vi "Read Tab Control Pane Dimension Width.vi"(8 "error in (no error)":errorcluster, 11 "TabControl.lvclass in":refnum<class "TabControl.lvclass">) -> (0 "error out":errorcluster, 2 "PaneWidth":u32, 3 "TabControl.lvclass out":refnum<class "TabControl.lvclass">)   [LabVIEW 2015, in "TabControl.lvclass"]
uses:
  TabControl.lvclass
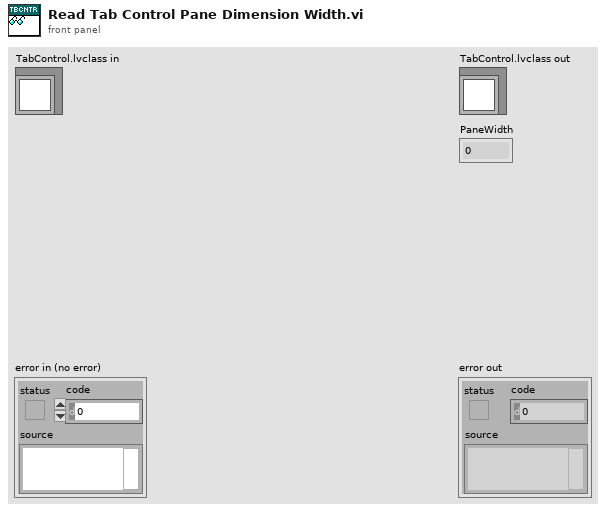
[diagram p1: front panel]
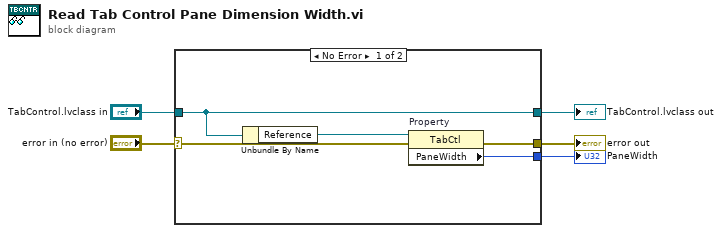
[diagram p0: block diagram]
diagram:
  n1 = case shown="No Error" "error in (no error)" {
    selector: "error in (no error)" -> [w6 w12]
    tunnel: [w9 w12] -> w4
    tunnel: [w8 w11] -> w2
    tunnel: "TabControl.lvclass in" -> [w8 w11]
    tunnel: [w10 _] -> w1
    frame No Error {
      n2 = Unbundle By Name(w8) -> ("Reference"=w7:refnum<vi>)
      n3 = property on="Property" class="TabCtl"(reference=w7, error in=w6) -> (error out=w9:errorcluster, "PaneWidth"=w10:u32)  [unwired: 1 out]
    }
    frame Error {
    }
  }
  "error out" <- w4
  "TabControl.lvclass out" <- w2
  "PaneWidth" <- w1
